vi "Temp1.vi"(6 "i":i32, 7 "w[i]":u32 format="0x%08x", 8 "h":u32, 9 "g":u32, 10 "f":u32, 11 "e":u32) -> (2 "Temp 1":u32)   [LabVIEW 2018, in "Crypto.lvlib" / "SHA-256.lvclass"]
uses:
  SHA-256.lvclass
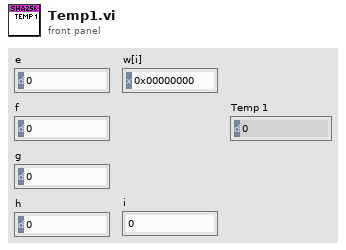
[diagram p1: front panel]
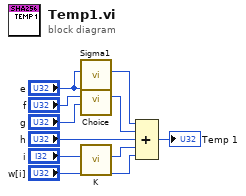
[diagram p0: block diagram]
diagram:
  n1 = call "Sigma1.vi"("Value"="e") -> ("Sigma 1"=w8:u32)  [unwired: 10 in]
  n2 = call "Choice.vi"("g"="g", "f"="f", "e"="e") -> ("Ch"=w7:u32)  [unwired: 8 in]
  n3 = call "K.vi"("i"="i") -> ("k[i]"=w9:u32)  [unwired: 10 in]
  n4 = Compound Arithmetic op=ADD(w8, w7, "h", w9, "w[i]") -> (→"Temp 1":u32)
